vi "4461 one board AOAI sync.vi"() -> ()   [LabVIEW 2020]
uses:
  <vilib>/DAQmx/write.llb/DAQmx Write (Analog 1D DBL 1Chan NSamp).vi
  <vilib>/DAQmx/read.llb/DAQmx Read (Analog 1D DBL 1Chan NSamp).vi
  <vilib>/DAQmx/create/channels.llb/DAQmx Create Channel (AO-Voltage-Basic).vi
  <vilib>/DAQmx/create/channels.llb/DAQmx Create Channel (AI-Voltage-Basic).vi
  <vilib>/DAQmx/configure/timing.llb/DAQmx Timing (Sample Clock).vi
  <vilib>/DAQmx/configure/trigger.llb/DAQmx Start Trigger (Digital Edge).vi
  <vilib>/DAQmx/miscellaneous.llb/DAQmx Fill In Error Info.vi
  <resource>/objmgr/daqmx.rc
  <vilib>/Analysis/NI_AALBase.lvlib
panel:
  out "Graph":dbl[](graph)
  in  "stop":bool
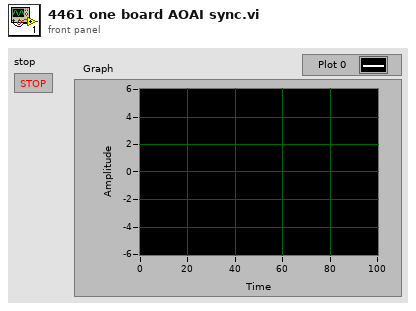
[diagram p1: front panel]
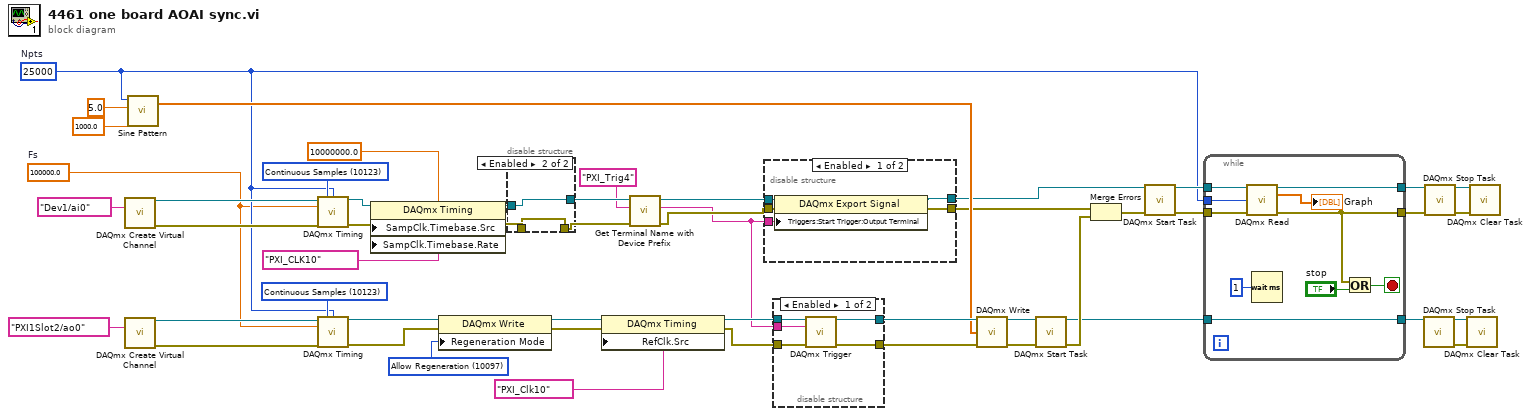
[diagram p0: block diagram]
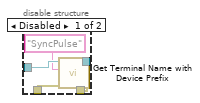
[diagram p2: hidden frame]
diagram:
  w16 = 100000.0  # Fs
  w42 = 10123 items=["Finite Samples"=10178, "Continuous Samples"=10123, "Hardware Timed Single Point"=12522] ("sample mode")
  w45 = 10097 items=["Allow Regeneration"=10097, "Do Not Allow Regeneration"=10158] ("RegenMode")
  w17 = 25000  # Npts
  w49 = 10123 items=["Finite Samples"=10178, "Continuous Samples"=10123, "Hardware Timed Single Point"=12522] ("sample mode")
  n1 = call-poly <vilib>:"DAQmx Create Virtual Channel.vi"("physical channels"=tag "Dev1/ai0") -> ("task out"=w51:refnum<k21>, "error out"=w50:errorcluster)  [unwired: 13 in]
  n2 = call-poly <vilib>:"DAQmx Create Virtual Channel.vi"("physical channels"=tag "PXI1Slot2/ao0") -> ("task out"=w48:refnum<k21>, "error out"=w44:errorcluster)  [unwired: 13 in]
  n3 = call <vilib>:"Sine Pattern.vi"("cycles"=1000.0, "amplitude"=5.0, "samples"=w17) -> ("Sinusoidal Pattern"=w23:dbl[])  [unwired: 1 in, 1 out]
  n4 = call-poly <vilib>:"DAQmx Timing.vi"("task/channels in"=w51, "sample mode"=w49, "samples per channel"=w17, "rate"=w16, "error in"=w50) -> ("task out"=w10:refnum<k21>, "error out"=w8:errorcluster)  [unwired: 9 in]
  n5 = call-poly <vilib>:"DAQmx Timing.vi"("task/channels in"=w48, "sample mode"=w42, "samples per channel"=w17, "rate"=w16, "error in"=w44) -> ("task out"=w46:refnum<k21>, "error out"=w47:errorcluster)  [unwired: 9 in]
  n6 = property class="DAQmx Timing"(reference=w10, error in=w8, "SampClk.Timebase.Src"=tag "PXI_CLK10" ("RefClk.Src"), "SampClk.Timebase.Rate"=10000000.0) -> (reference out=w9:refnum<k21>, error out=w7:errorcluster)
  n7 = property class="DAQmx Write"(reference=w46, error in=w47, "Regeneration Mode"=w45) -> (reference out=w41:refnum<k21>, error out=w40:errorcluster)
  n8 = disable-structure shown="Enabled" {
    disable-tunnel: w9 -> [w56 w58]
    disable-tunnel: w7 -> [w55 w57]
    disable-tunnel: [w54 w57] -> w4
    disable-tunnel: [w53 w58] -> w3
    frame Disabled {
      n9 = call "Get Terminal Name with Device Prefix.vi"("error in (no error)"=w55, "Local Terminal Name"="SyncPulse", "task/channels in"=w56) -> ("error out"=w54:errorcluster, "task out"=w53:refnum<k21>)  [unwired: 6 in, 1 out]
    }
    frame Enabled {
    }
  }
  n10 = property class="DAQmx Timing"(reference=w41, error in=w40, "RefClk.Src"=tag "PXI_Clk10") -> (reference out=w13:refnum<k21>, error out=w12:errorcluster)
  n11 = call "Get Terminal Name with Device Prefix.vi"("error in (no error)"=w4, "Local Terminal Name"="PXI_Trig4", "task/channels in"=w3) -> ("error out"=w15:errorcluster, "Terminal Name with Device Prefix"=w1:tag, "task out"=w14:refnum<k21>)  [unwired: 6 in]
  n12 = disable-structure shown="Enabled" {
    disable-tunnel: [w63 w65] -> w22
    disable-tunnel: [w62 w64] -> w21
    disable-tunnel: w15 -> [w61 w64]
    disable-tunnel: w14 -> [w60 w65]
    disable-tunnel: w1 -> [w59 _]
    frame Enabled {
      n13 = property class="DAQmx Export Signal"(reference=w60, error in=w61, "Triggers:Start Trigger:Output Terminal"=w59) -> (reference out=w63:refnum<k21>, error out=w62:errorcluster)
    }
    frame Disabled {
    }
  }
  n14 = disable-structure shown="Enabled" {
    disable-tunnel: [w70 w71] -> w27
    disable-tunnel: [w69 w72] -> w26
    disable-tunnel: w13 -> [w68 w72]
    disable-tunnel: w12 -> [w67 w71]
    disable-tunnel: w1 -> [w66 _]
    frame Enabled {
      n15 = call-poly <vilib>:"DAQmx Trigger.vi"("task/channels in"=w68, "source"=w66, "error in"=w67) -> ("task out"=w69:refnum<k21>, "error out"=w70:errorcluster)  [unwired: 11 in]
    }
    frame Disabled {
    }
  }
  n16 = call-poly <vilib>:"DAQmx Write.vi"("task/channels in"=w26, "data"=w23, "error in"=w27) -> ("task out"=w25:refnum<k21>, "error out"=w24:errorcluster)  [unwired: 10 in, 1 out]
  n17 = call <vilib>:"DAQmx Start Task.vi"("task/channels in"=w25, "error in"=w24) -> ("task out"=w35:refnum<k21>, "error out"=w39:errorcluster)  [unwired: 12 in]
  n18 = Merge Errors(w21, w39) -> (w38:errorcluster)
  n19 = call <vilib>:"DAQmx Start Task.vi"("task/channels in"=w22, "error in"=w38) -> ("task out"=w36:refnum<k21>, "error out"=w37:errorcluster)  [unwired: 12 in]
  n20 = while {
    tunnel: w37 -> [w78]
    tunnel: w36 -> [w79]
    tunnel: w35 -> [w80]
    tunnel: [w77] -> w34
    tunnel: [w73] -> w33
    tunnel: [w80] -> w32
    tunnel: w17 -> [w76]
    stop <- w74 stop-if-true
    n21 = call-poly <vilib>:"DAQmx Read.vi"("task/channels in"=w79, "number of samples per channel"=w76, "error in"=w78) -> ("task out"=w77:refnum<k21>, "data"=→"Graph":dbl[], "error out"=w73:errorcluster)  [unwired: 10 in]
    n22 = Wait (ms)(milliseconds to wait=u32 1) -> ()  [unwired: 1 out]
    n23 = Or(x=w73, y="stop") -> (x .or. y?=w74:bool)
  }
  n24 = call <vilib>:"DAQmx Stop Task.vi"("task/channels in"=w32) -> ("task out"=w29:refnum<k21>, "error out"=w28:errorcluster)  [unwired: 13 in]
  n25 = call <vilib>:"DAQmx Stop Task.vi"("task/channels in"=w34, "error in"=w33) -> ("task out"=w31:refnum<k21>, "error out"=w30:errorcluster)  [unwired: 12 in]
  n26 = call <vilib>:"DAQmx Clear Task.vi"("task in"=w29, "error in"=w28) -> ()  [unwired: 13 in, 1 out]
  n27 = call <vilib>:"DAQmx Clear Task.vi"("task in"=w31, "error in"=w30) -> ()  [unwired: 13 in, 1 out]
